vi "AMB_Dual_Interface_Find_Slaves.vi"(0 "ObjHandle in":u32, 1 "error in":errorcluster {"code" format="%.0x"}) -> (2 "ObjHandle out":u32, 3 "NumSlaves out":u8, 4 "Node Array out":cluster{"Address":u16, "Serial Number":i8[]}[](array[cluster]) {"Serial Number" format="%.0x"}, 5 "error out":errorcluster {"code" format="%.0x"})   [LabVIEW 2017]
doc: "This VI is a wrapper for the VIs 'AMB_TCP_Find_Slaves.vi' and 'AMB_CAN_Find_Slaves.vi'.\nIt uses the LabVIEW global 'AMB_Global.gbl.vi' to determine if communication is done over the CAN bus directly or if tunneling through TCP/IP is used.\n\nThe VI scans the CAN bus for connected nodes and list their node adress and serial number in an array (Node Array out) and the number of CAN nodes found (NumSlaves out).\nYou should have already setup the AMB with the AMB Setup VI."
uses:
  AMB_Global.gbl.vi
panel:
  # "Node Address"
  # "Serial Number"
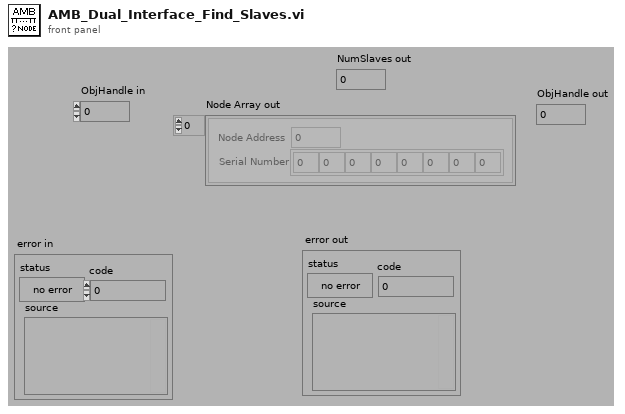
[diagram p1: front panel]
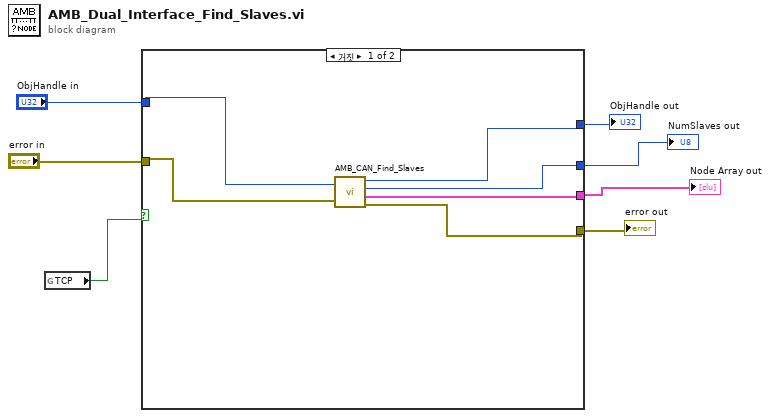
[diagram p0: block diagram]
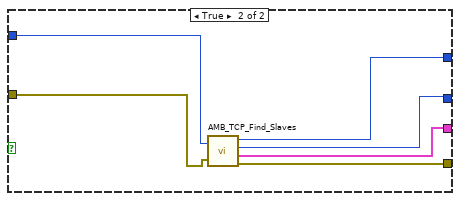
[diagram p2: hidden frame]
diagram:
  n1 = global read "AMB_Global.gbl.vi" "TCP"() -> (w7:bool)
  n2 = case shown="거짓" w7 {
    tunnel: "ObjHandle in" -> [w11 w17]
    tunnel: "error in" -> [w12 w19]
    tunnel: [w10 w16] -> w4
    tunnel: [w9 w14] -> w1
    tunnel: [w13 w18] -> w3
    tunnel: [w8 w15] -> w2
    frame False {
      n3 = call "AMB_CAN_Find_Slaves.vi"("ObjHandle in"=w11, "error in"=w12) -> ("ObjHandle out"=w10:u32, "NumSlaves out"=w8:u8, "Node Array out"=w9:cluster{"Address":u32, "Serial Number":i8[]}[], "error out"=w13:errorcluster)
    }
    frame True {
      n4 = call "AMB_TCP_Find_Slaves.vi"("ObjHandle In"=w17, "error in"=w19) -> ("ObjHandle Out"=w16:u32, "NumSlaves out"=w15:u8, "Node Array out"=w14:cluster{"Address":i8, "Serial Number":i8[]}[], "error out"=w18:errorcluster)
    }
  }
  "ObjHandle out" <- w4
  "error out" <- w3
  "NumSlaves out" <- w2
  "Node Array out" <- w1
